vi "UDP_send_v004.vi"() -> ()   [LabVIEW 2019]
panel:
  in  "Address selector":i32[](array[numeric])
  in  "Neuron ID":dbl(slide) scale=0.0..10.0
  in  "stop":bool
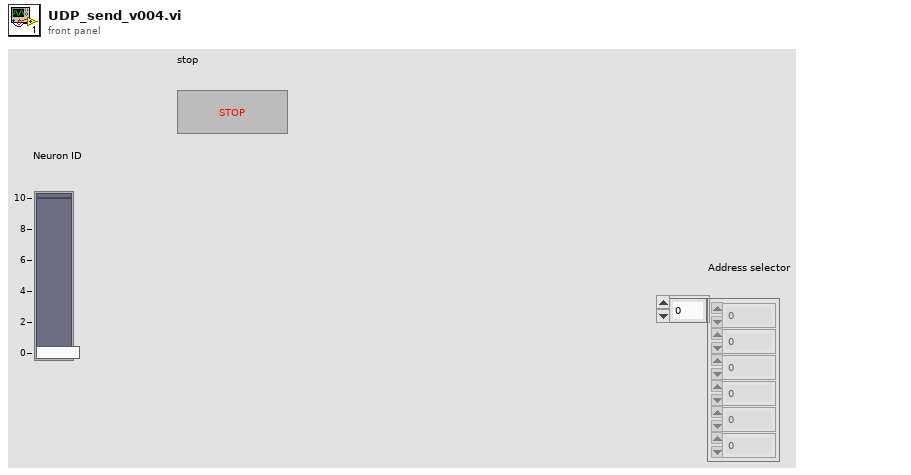
[diagram p1: front panel]
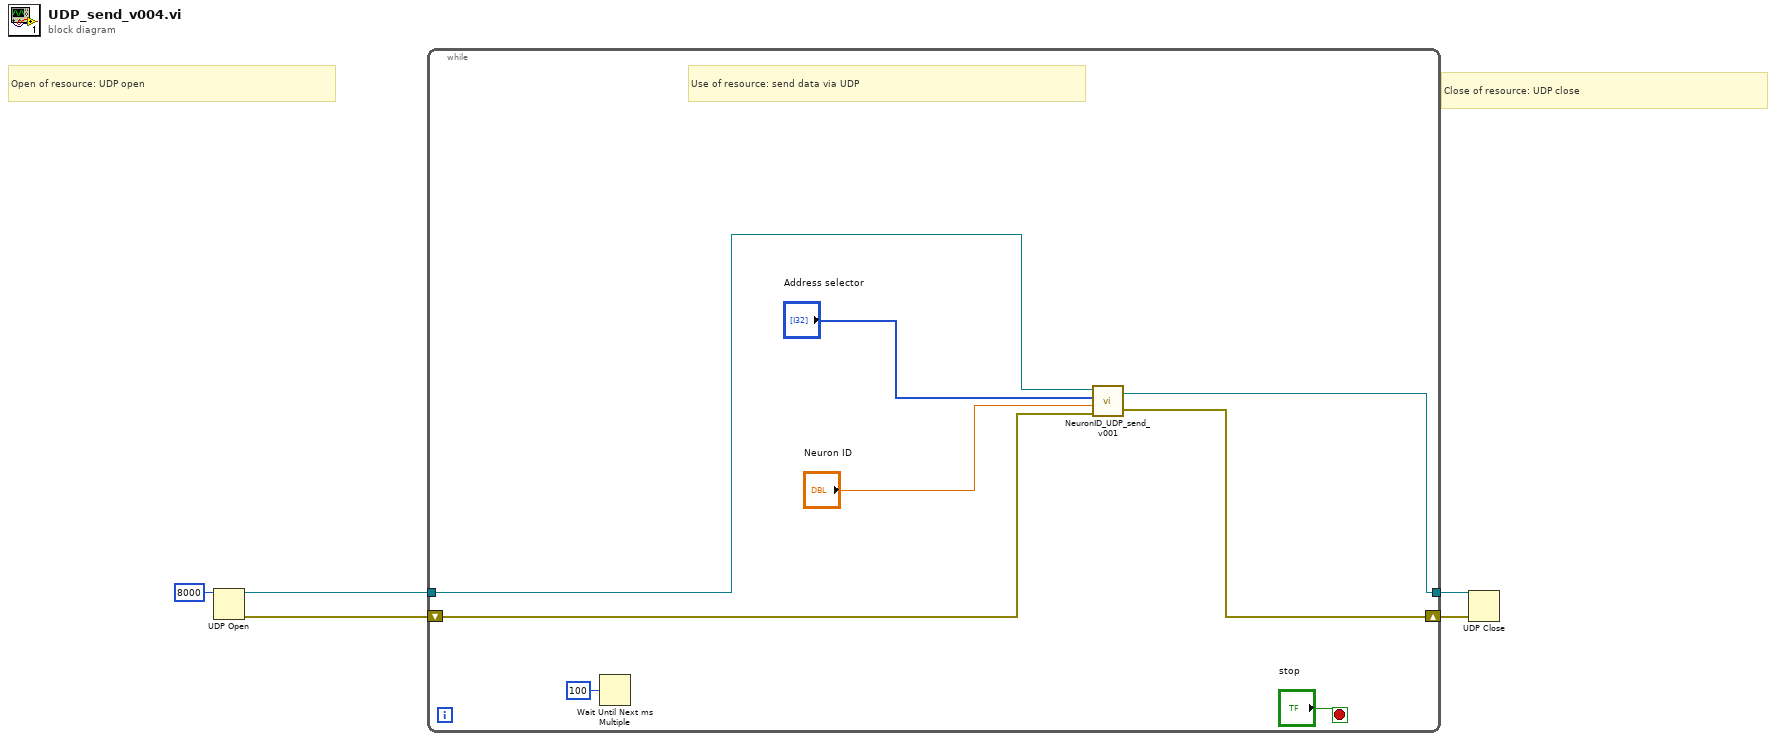
[diagram p0: block diagram]
diagram:
  # "Close of resource: UDP close"
  # "Open of resource: UDP open"
  n1 = UDP Open(11:u16 8000 ("port")) -> (port=w3:refnum<k16>, 0:w5:errorcluster)  [unwired: 4 in, 1 out]
  n2 = while {
    shift-right: [w10] -> w4
    shift-left: w5 -> [w11]
    tunnel: w3 -> [w9]
    tunnel: [w8] -> w2
    stop <- "stop" stop-if-true
    # "Use of resource: send data via UDP"
    n3 = Wait Until Next ms Multiple(millisecond multiple=u32 100) -> ()  [unwired: 1 out]
    n4 = call "NeuronID_UDP_send_v001.vi"("error in (no error)"=w11, "Neuron ID"="Neuron ID", "Address selector"="Address selector", "UDP Network Connection in"=w9) -> ("error out"=w10:errorcluster, "UDP Network Connection out"=w8:refnum<k16>)
  }
  n5 = UDP Close(connection ID=w2, 8:w4) -> ()  [unwired: 2 out]
